vi "On Client Certificate Requested.vi"(8 "error in (no error)":errorcluster, 10 "cluster":T2, 11 "WebView2 Event Filter Interface in":refnum<class "WebView2 Event Filter Interface.lvclass">) -> (0 "error out":errorcluster, 2 "Response":T1)   [LabVIEW 2025, in "WebView2.lvlib" / "WebView2 Event Filter Interface.lvclass"]
uses:
  WebView2 Event Filter Interface.lvclass
  WebView2 Control Object/Client Certificate Requested Event Data.ctl
  E:/Labview/LV 2023/PPL/PPL Builder/Libs/LV-WebView2/Source/Libs/Microsoft.Web.WebView2.Core.dll
  Libs/Microsoft.Web.WebView2.Core.dll
  WebView2 Control Object/WebView2 Control.lvclass
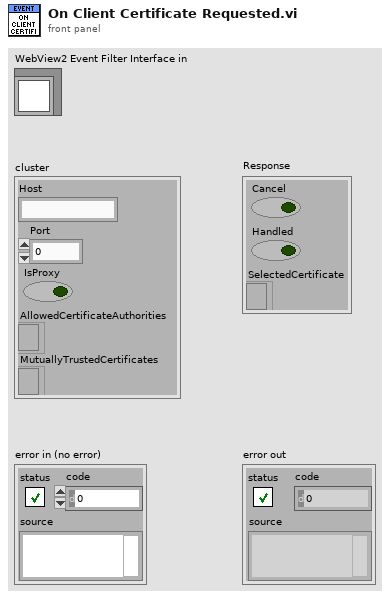
[diagram p1: front panel]
types:
  T1 = cluster{"Cancel":bool, "Handled":bool, "SelectedCertificate":refnum<k24>}
  T2 = typedef "WebView2.lvlib/WebView2 Control.lvclass/Client Certificate Requested Event Data.ctl" = cluster{"Host":string, "Port":i32, "IsProxy":bool, "AllowedCertificateAuthorities":refnum<k24>, "MutuallyTrustedCertificates":refnum<k24>}
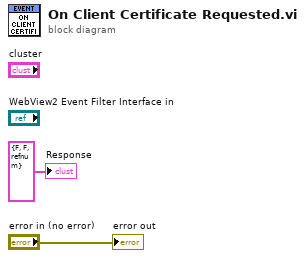
[diagram p0: block diagram]
diagram:
  "error out" <- "error in (no error)"
  "Response" <- T1 {"Cancel"=FALSE, "Handled"=FALSE, "SelectedCertificate"=refnum} ("Response")
